vi "myRIO_BRig_Host_endExp_filePath__announce.vi"() -> (2 "concatenated string":string)   [LabVIEW 2014]
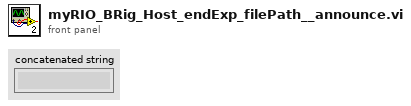
[diagram p1: front panel]
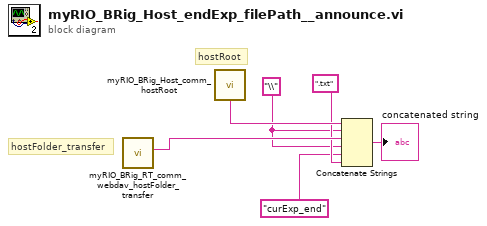
[diagram p0: block diagram]
diagram:
  w3 = "\\" ("string")
  # "hostFolder_transfer"
  # "hostRoot"
  n1 = call "myRIO_BRig_RT_comm_webdav_hostFolder_transfer.vi"() -> ("output_HostFolder"=w5:string)  [unwired: 11 in]
  n2 = call "myRIO_BRig_Host_comm_hostRoot.vi"() -> ("output_hostRoot"=w6:string)  [unwired: 11 in]
  n3 = Concatenate Strings(w6, w3, w5, w3, "curExp_end" ("string"), ".txt" ("string")) -> (→"concatenated string":string)
